vi "Zcam.vi"() -> ()   [LabVIEW 2014]
uses:
  <vilib>/userdefined/High Color/VBAIInterface.ctl
  <vilib>/vision/Vision Builder AI/API.llb/VBAI Interface - Get Inspection Image (By Name).vi
panel:
  out "Image Dst Out":T1(plugin-control)
  in  "stop":bool
  in  "Session In":T2
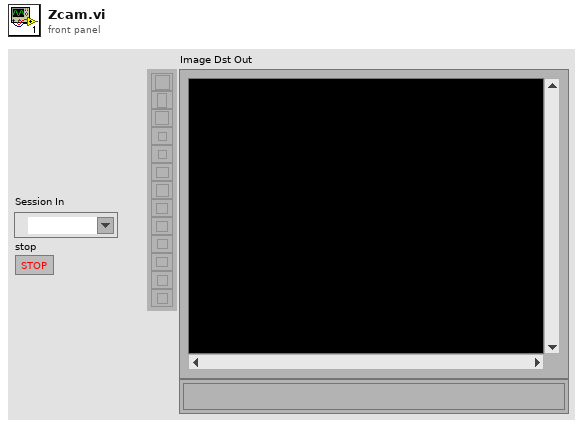
[diagram p1: front panel]
types:
  T1 = typedef "IMAQ Image.ctl" = refnum<image>
  T2 = typedef "VBAIInterface.ctl" = refnum<k21>
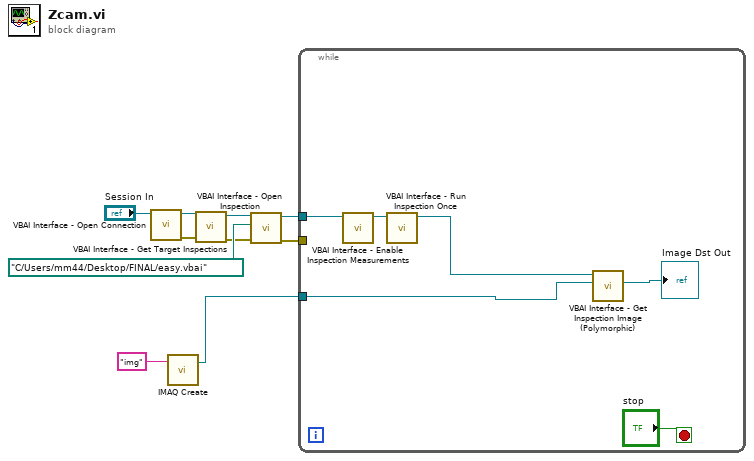
[diagram p0: block diagram]
diagram:
  n1 = call <vilib>:"VBAI Interface - Open Connection.vi"("Session In"="Session In") -> ("error out"=w5:errorcluster, "Session Out"=w9:T2)  [unwired: 9 in]
  n2 = call "IMAQ Create"("Image Name"="img") -> ("New Image"=w1:T1)  [unwired: 4 in, 1 out]
  n3 = call <vilib>:"VBAI Interface - Get Target Inspections.vi"("error in"=w5, "Session In"=w9) -> ("error out"=w4:errorcluster, "Session Out"=w8:T2)  [unwired: 7 in, 1 out]
  n4 = call <vilib>:"VBAI Interface - Open Inspection.vi"("error in"=w4, "Path"=path "C:/Users/mm44/Desktop/FINAL/easy.vbai", "Session In"=w8) -> ("error out"=w3:errorcluster, "Session Out"=w7:T2)  [unwired: 7 in]
  n5 = while {
    tunnel: w7 -> [w16]
    tunnel: w3 -> [_]
    tunnel: w1 -> [w11]
    stop <- "stop" stop-if-true
    n6 = call <vilib>:"VBAI Interface - Enable Inspection Measurements.vi"("Session In"=w16) -> ("Session Out"=w15:T2)  [unwired: 9 in, 1 out]
    n7 = call <vilib>:"VBAI Interface - Run Inspection Once.vi"("Session In"=w15) -> ("Session Out"=w14:T2)  [unwired: 9 in, 1 out]
    n8 = call-poly <vilib>:"VBAI Interface - Get Inspection Image (Polymorphic).vi"("Image Dest"=w11, "Session In"=w14) -> ("Image Dst Out"=→"Image Dst Out":T1)  [unwired: 6 in, 3 out]
  }
